vi "CSM-TrialLicWatermark.vi"(6 "Trial(600s)":dbl=600.0, 8 "error in (no error)":errorcluster, 11 "TrialLicWatermark":refnum<vi>) -> (0 "error out":errorcluster, 2 "time up?":bool, 3 "passed":dbl)   [LabVIEW 2017]
uses:
  <vilib>/Utility/miscctls.llb/LVPositionTypeDef.ctl
  <vilib>/Utility/miscctls.llb/LVRectTypeDef.ctl
  Communicable State Machine.lvlib
panel:
  in  "Watermark":string
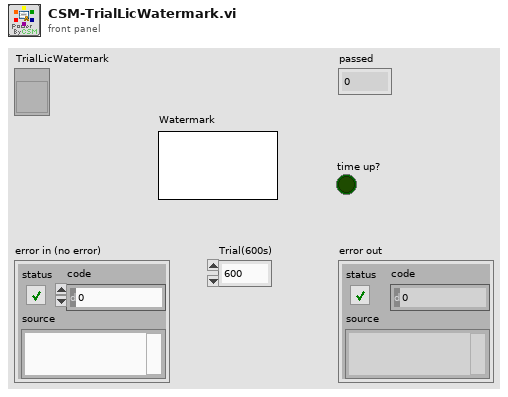
[diagram p1: front panel]
types:
  T1 = enum8{"Enabled", "Disabled", "Disabled and Grayed Out"}
  T2 = typedef "LVRectTypeDef.ctl" = cluster{"Left":i16, "Top":i16, "Right":i16, "Bottom":i16}
  T3 = typedef "LVPositionTypeDef.ctl" = cluster{"Left":i32, "Top":i32}
  T4 = typedef "LVBoundsTypeDef.ctl" = cluster{"Width":u32, "Height":u32}
  T5 = cluster{"left":i16, "top":i16, "right":i16, "bottom":i16}
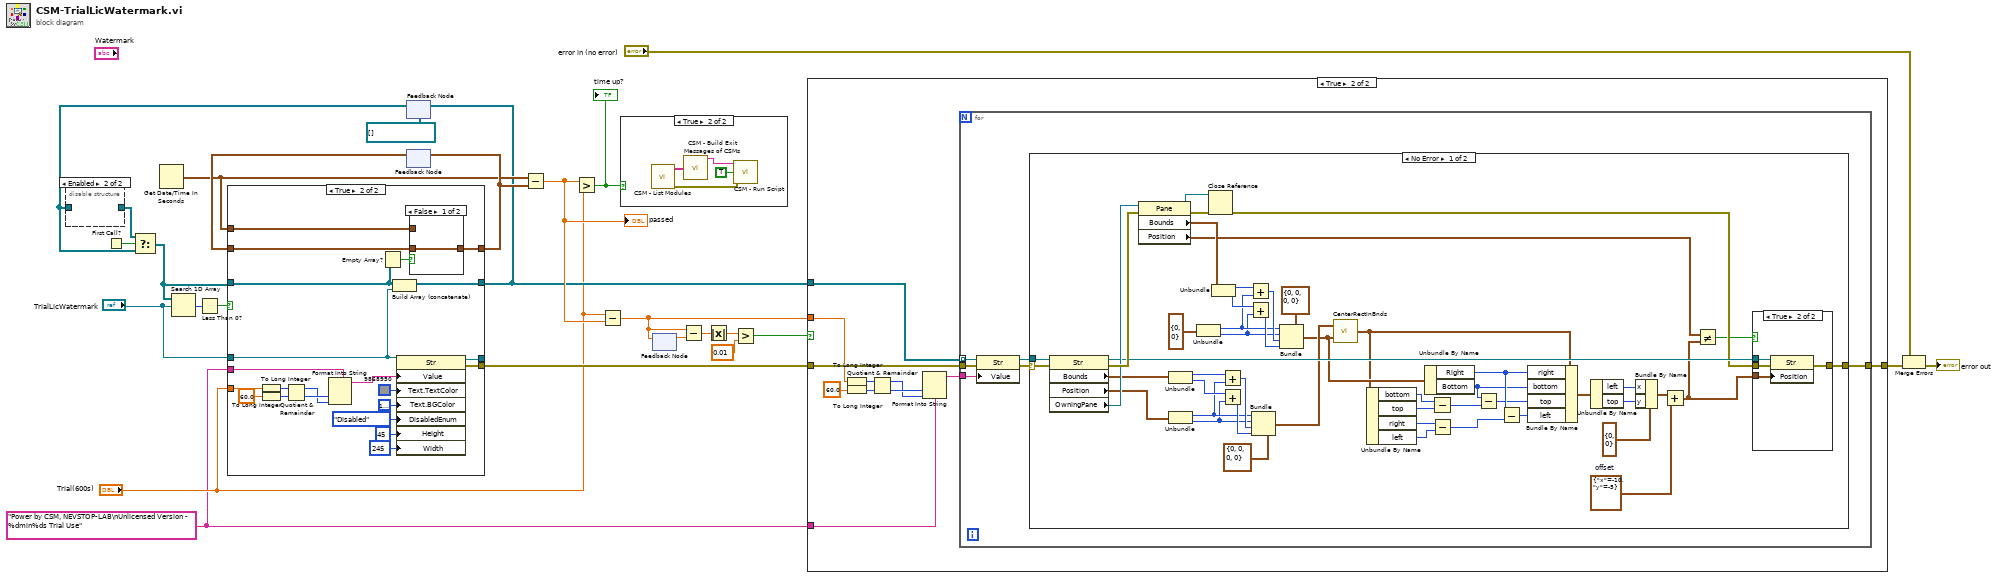
[diagram p0: block diagram]
diagram:
  w1 = "Power by CSM, NEVSTOP-LAB\nUnlicensed Version - %dmin%ds Trial Use" ("Value")
  n1 = First Call?() -> (First Call?: T/F=w23:bool)
  n2 = Get Date/Time In Seconds() -> (seconds since 1Jan1904=w16:timestamp)
  n3 = feedback #1(refnum<vi>[] [] ("Prompt")) -> (w19:refnum<vi>[])
  n4 = disable-structure shown="Enabled" {
    disable-tunnel: [w27 _] -> w20
    disable-tunnel: w19 -> [w27 _]
    frame Disabled {
    }
    frame Enabled {
    }
  }
  n5 = Select(t=w20, s=w23, f=w19) -> (s? t:f=w21:refnum<vi>[])
  n6 = Search 1D Array(1D array=w21, element="TrialLicWatermark") -> (index of element=w25:i32)  [unwired: 1 in]
  n7 = Less Than 0?(x=w25) -> (x < 0?=w26:bool)
  n8 = feedback #2() -> (w18:timestamp)  [unwired: 1 in]
  n9 = case shown="True" w26 {
    tunnel: "TrialLicWatermark" -> [w29 w47]
    tunnel: [w29 w52] -> _
    tunnel: [_ w48] -> w5
    tunnel: w21 -> [w30 w45]
    tunnel: [w30 w46] -> w12
    tunnel: [w28 w43] -> w17
    tunnel: w18 -> [w28 w42]
    tunnel: w16 -> [_ w41]
    tunnel: w1 -> [_ w38]
    tunnel: "Trial(600s)" -> [_ w35]
    frame False {
    }
    frame True {
      n10 = To Long Integer(number=w35) -> (32bit integer=w33:i32)
      n11 = To Long Integer(number=60.0 ("y")) -> (32bit integer=w34:i32)
      n12 = Quotient & Remainder(x=w33, y=w34) -> (x-y*floor(x/y)=w31:i32, floor(x/y)=w32:i32)
      n13 = Format Into String(format string=w38, w32, w31) -> (resulting string=w37:string)  [unwired: 2 in, 1 out]
      n14 = Empty Array?(array=w45) -> (empty?=w44:bool)
      n15 = Build Array (concatenate)(w45, w47) -> (w46:refnum<vi>[])
      n16 = property class="Str"(reference=w47, "Value"=w37, "Text.TextColor"=u32 9868950 ("Text.Text Colors:Text Color"), "Text.BGColor"=u32 16777216 ("Text.Text Colors:Text Color"), "DisabledEnum"=T1."Disabled" ("Disabled"), "Height"=u32 45 ("Size:Height"), "Width"=u32 245 ("Size:Width")) -> (reference out=w52:refnum<vi>, error out=w48:errorcluster)  [unwired: 1 in]
      n17 = case shown="False" w44 {
        tunnel: [w53 w54] -> w43
        tunnel: w42 -> [w53 _]
        tunnel: w41 -> [_ w54]
        frame False {
        }
        frame True {
        }
      }
    }
  }
  n18 = feedback-in #1(w12) -> ()
  n19 = feedback-in #2(w17) -> ()
  n20 = Subtract(x=w16, y=w17) -> (x-y=w13:dbl)
  "passed" <- w13
  n21 = Greater?(x=w13, y="Trial(600s)") -> (0:w15:bool)
  "time up?" <- w15
  n22 = Subtract(x="Trial(600s)", y=w13) -> (x-y=w10:dbl)
  n23 = case shown="True" w15 {
    frame False {
    }
    frame True {
      n24 = call "CSM - List Modules.vi"() -> ("error out"=w58:errorcluster, "Module Names"=w56:string[])  [unwired: 10 in]
      n25 = call "CSM - Build Exit Messages of CSMs.vi"("CSMs"=w56) -> ("States"=w57:string)  [unwired: 14 in]
      n26 = call "CSM - Run Script.vi"("CSM Scripts"=w57, "Continue If Error? (F)"=TRUE, "error in (no error)"=w58) -> ()  [unwired: 10 in, 3 out]
    }
  }
  n27 = feedback #3() -> (w11:dbl)  [unwired: 1 in]
  n28 = feedback-in #3(w10) -> ()
  n29 = Subtract(x=w10, y=w11) -> (x-y=w7:dbl)
  n30 = Absolute Value(x=w7) -> (abs(x)=w6:dbl)
  n31 = Greater?(x=w6, y=0.01) -> (0:w8:bool)
  n32 = case shown="True" w8 {
    tunnel: w5 -> [w59 w70]
    tunnel: [w59 w69] -> w14
    tunnel: w12 -> [_ w67]
    tunnel: w10 -> [_ w62]
    tunnel: w1 -> [_ w66]
    frame False {
    }
    frame True {
      n33 = To Long Integer(number=w62) -> (32bit integer=w63:i32)
      n34 = To Long Integer(number=60.0 ("y")) -> (32bit integer=w64:i32)
      n35 = Quotient & Remainder(x=w63, y=w64) -> (x-y*floor(x/y)=w60:i32, floor(x/y)=w61:i32)
      n36 = Format Into String(format string=w66, w61, w60) -> (resulting string=w68:string)  [unwired: 2 in, 1 out]
      n37 = for {
        tunnel: w68 -> [w75]
        tunnel: w70 -> [w76]
        tunnel: [w71] -> w69
        tunnel: w67 -> [w74] mode=indexing
        n38 = property class="Str"(reference=w74, error in=w76, "Value"=w75) -> (reference out=w73:refnum<vi>, error out=w72:errorcluster)
        n39 = case shown="No Error" w72 {
          selector: w72 -> [w114 w131]
          tunnel: w73 -> [w116 _]
          tunnel: [w115 w131] -> w71
          frame No Error {
            w109 = cluster{"x":i32, "y":i32} {"x"=-10, "y"=-5}  # offset
            n40 = property on="Property Node" class="Str"(reference=w116, error in=w114) -> (reference out=w122:refnum<vi>, error out=w124:errorcluster, "Bounds"=w117:T4, "Position"=w118:T3, "OwningPane"=w123:refnum<vi>)
            n41 = property on="Property Node" class="Pane"(reference=w123, error in=w124) -> (reference out=w110:refnum<vi>, error out=w125:errorcluster, "Bounds"=w119:T4, "Position"=w79:T3)
            n42 = Unbundle(w117) -> ("Width"=w99:u32, "Height"=w98:u32)
            n43 = Unbundle(w118) -> ("Left"=w95:i32, "Top"=w94:i32)
            n44 = Unbundle(T3 {"Left"=0, "Top"=0} ("Position")) -> ("Left"=w102:i32, "Top"=w101:i32)
            n45 = Close Reference(reference=w110, error in (no error)=w125) -> (error out=w111:errorcluster)
            n46 = Unbundle(w119) -> ("Width"=w106:u32, "Height"=w105:u32)
            n47 = Add(x=w99, y=w95) -> (x+y=w97:u32)
            n48 = Add(x=w98, y=w94) -> (x+y=w96:u32)
            n49 = Add(x=w106, y=w102) -> (x+y=w104:u32)
            n50 = Add(x=w105, y=w101) -> (x+y=w103:u32)
            n51 = Bundle(cluster=T2 {"Left"=0, "Top"=0, "Right"=0, "Bottom"=0} ("Windows Bounds"), "Left"=w95, "Top"=w94, "Right"=w97, "Bottom"=w96) -> (w121:T2)
            n52 = Bundle(cluster=T2 {"Left"=0, "Top"=0, "Right"=0, "Bottom"=0} ("Windows Bounds"), "Left"=w102, "Top"=w101, "Right"=w104, "Bottom"=w103) -> (w120:T2)
            n53 = call <vilib>:"CenterRectInBnds.vi"("bounds"=w120, "rect"=w121) -> ("centered rect"=w86:T5)
            n54 = Unbundle By Name(w86) -> ("bottom"=w83:i16, "top"=w84:i16, "right"=w89:i16, "left"=w90:i16)
            n55 = Unbundle By Name(w120) -> ("Right"=w91:i16, "Bottom"=w88:i16)
            n56 = Subtract(x=w83, y=w84) -> (x-y=w85:i16)
            n57 = Subtract(x=w89, y=w90) -> (x-y=w92:i16)
            n58 = Subtract(x=w88, y=w85) -> (x-y=w87:i16)
            n59 = Subtract(x=w91, y=w92) -> (x-y=w93:i16)
            n60 = Bundle By Name(cluster=w86, "right"=w91, "bottom"=w88, "top"=w87, "left"=w93) -> (w113:T5)
            n61 = Unbundle By Name(w113) -> ("left"=w81:i16, "top"=w82:i16)
            n62 = Bundle By Name(cluster=cluster{"x":i32, "y":i32} {"x"=0, "y"=0} ("Point"), "x"=w81, "y"=w82) -> (w112:cluster{"x":i32, "y":i32})
            n63 = Add(x=w112, y=w109) -> (x+y=w78:cluster{"x":i32, "y":i32})
            n64 = Not Equal?(x=w79, y=w78) -> (x != y?=w77:bool)
            n65 = case shown="True" w77 {
              tunnel: w122 -> [_ w130]
              tunnel: [w126 w129] -> w115
              tunnel: w111 -> [w126 w128]
              tunnel: w78 -> [_ w127]
              frame False {
              }
              frame True {
                n66 = property on="Property Node" class="Str"(reference=w130, error in=w128, "Position"=w127) -> (error out=w129:errorcluster)  [unwired: 1 out]
              }
            }
          }
          frame Error {
          }
        }
      }
    }
  }
  n67 = Merge Errors("error in (no error)", w14) -> (→"error out":errorcluster)
